vi "截屏.vi"() -> ()   [LabVIEW 2013]
uses:
  <vilib>/printing/EasyPrintingControls.llb/contents.ctl
  <vilib>/printing/EasyPrintingControls.llb/report_type.ctl
  <vilib>/Utility/NIReport.llb/NI_report.lvclass
  <vilib>/printing/EasyPrinting.llb/Easy Print VI Panel or Documentation (path).vi
  <vilib>/Utility/NIReport.llb/NI_ReportGenerationCore.lvlib
panel:
  in  "数据保存":bool
  out "error out 4":errorcluster caption="错误输出"
  in  "产品ID":string
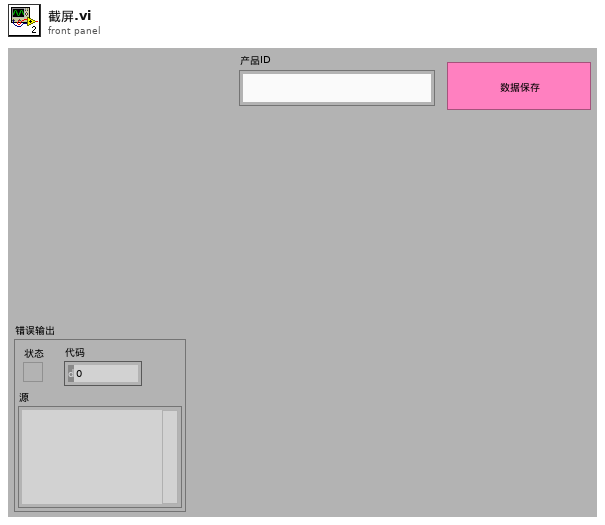
[diagram p1: front panel]
types:
  T1 = typedef "NI_ReportGenerationCore.lvlib/report_type.ctl" = u16
  T2 = typedef "NI_ReportGenerationCore.lvlib/contents.ctl" = u16
diagram:
  n1 = case shown="真" "数据保存" {
    frame False {
    }
    frame True {
      w10 = T1 2 items=["快速打印", "标准报表", "HTML", "双字节", "Excel"] ("report type (Quick Print)")
      w11 = T2 1 items=["完整前面板", "前面板可见部分", "图标、说明、前面板和程序框图", "说明信息: 使用前面板", "说明信息: 作为子VI使用", "说明信息: 完整", "说明信息: 自定义"] ("contents (complete front panel)")
      n2 = local read "产品ID"() -> (w6:string)
      n3 = Current VI's Path() -> (path=w12:path)
      n4 = Concatenate Strings(w6, ".BMP" ("产品ID")) -> (w5:string)
      n5 = call-poly <vilib>:"Easy Print VI Panel or Documentation.vi"("report type (Quick Print)"=w10, "contents (complete front panel)"=w11, "VI path"=w12) -> ("error out"=w3:errorcluster, "report out"=w9:refnum<class "NI_report.lvclass">)  [unwired: 1 in, 6 out]
      n6 = Build Path(base path=path "C:/Users/Q13038/Desktop" ("基路径"), name or relative path=w5) -> (appended path=w4:path)
      n7 = call-dynamic "Save Report to File.vi"("report in"=w9, "report file path"=w4, "error in (no error)"=w3) -> ("error out"=→"error out 4":errorcluster)  [unwired: 2 in, 10 out]
    }
  }
